vi "GPS -Evnt On Position Change.vi"(4 "User Parameter":variant, 5 "Event Data":cluster{"point":refnum<k24>}, 6 "Control Ref":refnum<k24>, 7 "Event Common Data":T1) -> ()   [LabVIEW 2019]
uses:
  \\mac\Dropbox/gmap.net/GMAP.NET 8.6/data/GMap.NET.WindowsForms.dll
  data/GMap.NET.WindowsForms.dll
  \\mac\Dropbox/gmap.net/GMAP.NET 8.6/data/GMap.NET.Core.dll
  data/GMap.NET.Core.dll
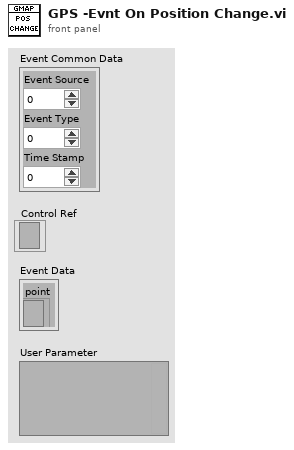
[diagram p1: front panel]
types:
  T1 = cluster{"Event Source":i32, "Event Type":u32, "Time Stamp":u32}
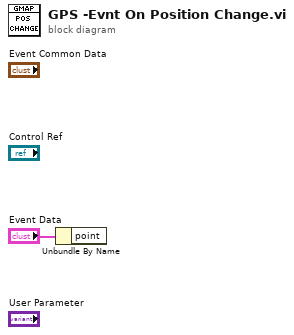
[diagram p0: block diagram]
diagram:
  n1 = Unbundle By Name("Event Data") -> ()  [unwired: 1 out]
